vi "FormatDMAelement_4.vi"(8 "valid in":bool, 11 "Data in":fxp<+/-,16,14>[](array[numeric])=[0.0, 0.0, 0.0, 0.0, 0.0, 0.0, 0.0, 0.0]) -> (0 "valid out":bool, 2 "Element2":u64, 3 "Element1":u64)   [LabVIEW 2013]
uses:
  <vilib>/rvi/FXPMathLib/FxpInterpret/XNode/nifxpmath_Interpret.xnode
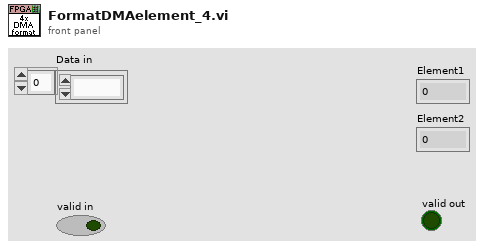
[diagram p1: front panel]
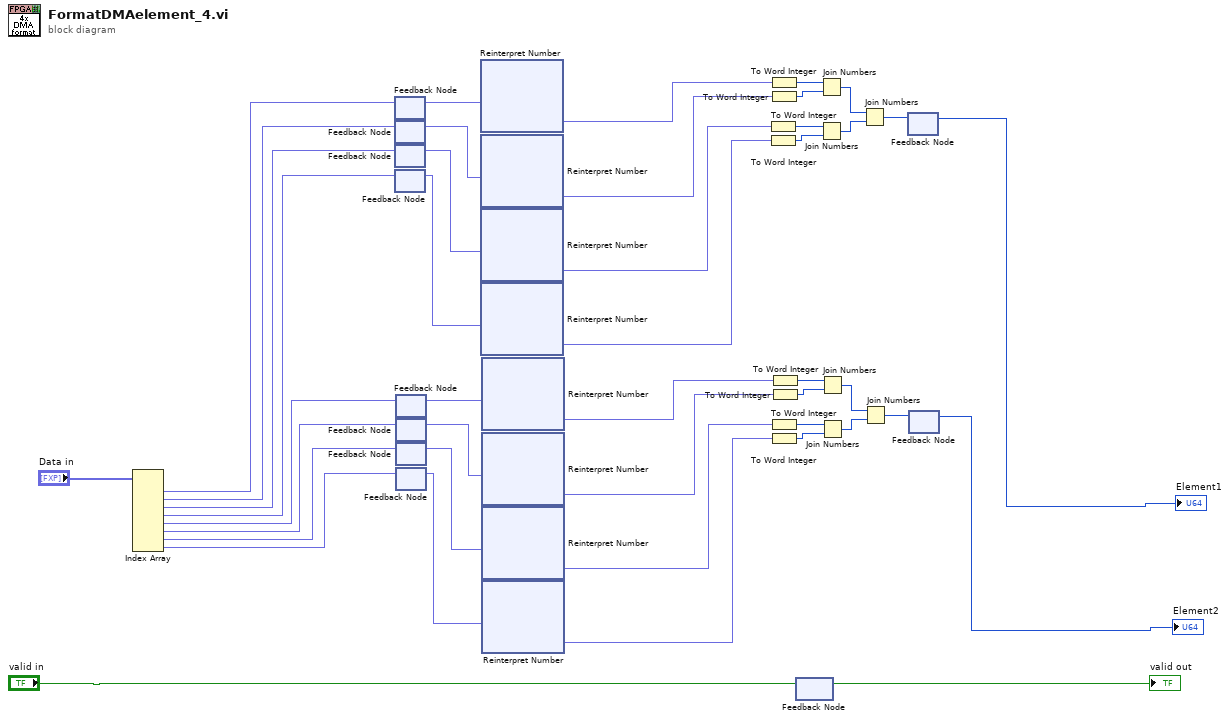
[diagram p0: block diagram]
diagram:
  n1 = Index Array(array="Data in") -> (element #1=w9:fxp<+/-,16,14>, element #2=w8:fxp<+/-,16,14>, element #3=w7:fxp<+/-,16,14>, element #4=w6:fxp<+/-,16,14>, element #5=w5:fxp<+/-,16,14>, element #6=w4:fxp<+/-,16,14>, element #7=w3:fxp<+/-,16,14>, element #8=w2:fxp<+/-,16,14>)  [unwired: 8 in]
  n2 = feedback #1() -> (w32:fxp<+/-,16,14>)  [unwired: 1 in]
  n3 = feedback-in #1(w9) -> ()
  n4 = feedback #2() -> (w30:fxp<+/-,16,14>)  [unwired: 1 in]
  n5 = feedback-in #2(w8) -> ()
  n6 = feedback #3() -> (w29:fxp<+/-,16,14>)  [unwired: 1 in]
  n7 = feedback-in #3(w7) -> ()
  n8 = feedback #4() -> (w28:fxp<+/-,16,14>)  [unwired: 1 in]
  n9 = feedback-in #4(w6) -> ()
  n10 = feedback #5() -> (w16:fxp<+/-,16,14>)  [unwired: 1 in]
  n11 = feedback-in #5(w5) -> ()
  n12 = feedback #6() -> (w18:fxp<+/-,16,14>)  [unwired: 1 in]
  n13 = feedback-in #6(w4) -> ()
  n14 = feedback #7() -> (w19:fxp<+/-,16,14>)  [unwired: 1 in]
  n15 = feedback-in #7(w3) -> ()
  n16 = feedback #8() -> (w20:fxp<+/-,16,14>)  [unwired: 1 in]
  n17 = feedback-in #8(w2) -> ()
  n18 = xnode "Reinterpret Number"("x"=w32) -> ("y"=w31:fxp<+/-,16,16>)
  n19 = xnode "Reinterpret Number"("x"=w30) -> ("y"=w27:fxp<+/-,16,16>)
  n20 = xnode "Reinterpret Number"("x"=w29) -> ("y"=w26:fxp<+/-,16,16>)
  n21 = xnode "Reinterpret Number"("x"=w28) -> ("y"=w25:fxp<+/-,16,16>)
  n22 = xnode "Reinterpret Number"("x"=w16) -> ("y"=w17:fxp<+/-,16,16>)
  n23 = xnode "Reinterpret Number"("x"=w18) -> ("y"=w21:fxp<+/-,16,16>)
  n24 = xnode "Reinterpret Number"("x"=w19) -> ("y"=w22:fxp<+/-,16,16>)
  n25 = xnode "Reinterpret Number"("x"=w20) -> ("y"=w1:fxp<+/-,16,16>)
  n26 = To Word Integer(number=w26) -> (16bit integer=w36:i16)
  n27 = To Word Integer(number=w25) -> (16bit integer=w35:i16)
  n28 = To Word Integer(number=w31) -> (16bit integer=w37:i16)
  n29 = To Word Integer(number=w27) -> (16bit integer=w38:i16)
  n30 = To Word Integer(number=w22) -> (16bit integer=w12:i16)
  n31 = To Word Integer(number=w1) -> (16bit integer=w13:i16)
  n32 = To Word Integer(number=w17) -> (16bit integer=w11:i16)
  n33 = To Word Integer(number=w21) -> (16bit integer=w10:i16)
  n34 = feedback #9() -> (→"valid out":bool)  [unwired: 1 in]
  n35 = feedback-in #9("valid in") -> ()
  n36 = Join Numbers(hi=w37, lo=w38) -> ((hi.lo)=w34:u32)
  n37 = Join Numbers(hi=w36, lo=w35) -> ((hi.lo)=w33:u32)
  n38 = Join Numbers(hi=w11, lo=w10) -> ((hi.lo)=w14:u32)
  n39 = Join Numbers(hi=w12, lo=w13) -> ((hi.lo)=w15:u32)
  n40 = Join Numbers(hi=w34, lo=w33) -> ((hi.lo)=w24:u64)
  n41 = Join Numbers(hi=w14, lo=w15) -> ((hi.lo)=w23:u64)
  n42 = feedback #10() -> (→"Element1":u64)  [unwired: 1 in]
  n43 = feedback-in #10(w24) -> ()
  n44 = feedback #11() -> (→"Element2":u64)  [unwired: 1 in]
  n45 = feedback-in #11(w23) -> ()
